vi "OpticsTester.vi"() -> ()   [LabVIEW 2024]
uses:
  <vilib>/SmarAct/SmarActCTL/SA_CTL.lvclass
  <vilib>/Platform/TimedLoop/XDataNode/timing_clust.ctl
  <vilib>/Platform/TimedLoop/XDataNode/nitl_modes.ctl
  <vilib>/Platform/TimedLoop/XDataNode/wakeup.ctl
  <vilib>/Utility/miscctls.llb/LVMajorAndMinorColorsTypeDef.ctl
  <vilib>/Analysis/1siggen.llb/Ramp Pattern by Delta.vi
  <vilib>/platform/TimedLoop/XDataNode/XDataNode.xnode
  <vilib>/Analysis/NI_AALBase.lvlib
  <userlib>/_OpenG.lib/time/time.llb/openg_time.lvlib
  <vilib>/Analysis/NI_AALPro.lvlib
  <vilib>/Platform/TimedLoop/XDataNode/XDNodeRunTimeDep.lvlib
  <instrlib>/Keithley 648X Series/Keithley 648X Series.lvlib
panel:
  in  "Measurement Time":dbl=6.0
  out "PicoAmmeter_VISA":refnum<visa-resource-name>
  in  "Oversample":i32=1000 min=1 max=4096
  out "Ref":dbl[](array[numeric])
  out "SweepData":dbl[][](array[numeric])
  in  "Exit":bool
  out "PositionerStatus":T1={"Moving"=FALSE, "CL Active"=FALSE, "Calibrating"=FALSE, "Referencing"=FALSE, "Delayed Move"=FALSE, "Sensor Present"=TRUE, "Is Calibrated"=TRUE, "Is Referenced"=TRUE, "End Stop"=FALSE, "Ranger Limit"=FALSE, "Following Limit"=FALSE, "Movement Fail"=FALSE, "Is Streaming"=FALSE, "Overload"=FALSE, "Over Temp"=FALSE, "Reference Mark"=FALSE, "Is Phased"=FALSE, "Positioner Fault"=FALSE, "Amplifier Enabled"=TRUE, "In Position"=FALSE, "Brake Enabled"=FALSE}
  out "ChannelState":i32=262368 format="%x"
  in  "Measurement Mode":T2(tab)=enum."Stage Calibration"
  in  "Device Locator":string(combo)="network:sn:MCS2-00005242"
  in  "findDevices":bool caption="Find Devices"
  in  "connect":bool
  out "connected":bool=TRUE
  out "Error Out":errorcluster
  in  "calibrate":bool
  in  "reference":bool
  in  "moveValue":i64=-10400000000 caption="Move Abs (µm)"
  in  "moveMode":u16(ring) caption="Move Mode" items=["CL_ABS", "CL_REL", "SCAN_ABS", "SCAN_REL", "STEP"]
  in  "move":bool
  in  "actuatorMode":enum32{"0", "1"}(radio)
  out "MCSChannel":i8
  out "Position (µm)":dbl=-7999576013.0
  in  "MoveStage":bool
  in  "Move To (mm)":dbl min=-13.5 max=13.5
  in  "Enable":bool=TRUE
  in  "Positioner\n Delay (ms)":u16(ring)=2 items=["1", "2", "5", "10", "20", "50", "100", "200", "500"]
  in  "Delay(mS)":u32=5
  out "Elapsed (ms)":dbl=6.0
  out "Waveform Chart":dbl(graph)=-7999.576013
  out "Peak-to-Peak (µm)":dbl=0.0026870000001508743 format="%^.4g"
  out "rms (µm)":dbl=-2.7284841053187847e-12 format="%^.4g"
  in  "Recalibrate":bool
  out "Calibration":cluster{"Array":dbl[], "Array":dbl[]}(graph)
  in  "Stage\nCal":dbl[][](array[numeric])=[[1020.0, -8440.0], [1100.0, -6120.0], [1200.0, -3330.0], [1300.0, -530.0], [1400.0, 2280.0], [1500.0, 5160.0], [1600.0, 8630.0]]
  out "slope":dbl
  out "intercept":dbl
  in  "Clear_Static":bool
  out "PhotoCurrent":dbl(graph)
  in  "Grid":bool
  in  "SetSample":bool
  in  "SetRef":bool
  in  "Dark Level":dbl
  out "End(nm)":dbl
  out "Start(nm)":dbl
  out "Sweep":cluster{"Ramp Pattern":dbl[], dbl[]}(graph)
  in  "Go":bool
  in  "Step(µm)":dbl=10.0 min=1.0 max=2000.0 step=1.0
  in  "Finish (mm)":dbl=-8.0 min=-12.0 max=12.0 step=1.0
  in  "Start (mm)":dbl=-12.0 min=-12.0 max=12.0 step=1.0
  in  "milliseconds\n to wait":u32 max=1000
  out "Elapsed(s)":dbl=32.049
  out "Cursor\nlambda":dbl
  out "samples":i32
  out "Step(nm)":dbl
  out "Reference":cluster{"Ramp Pattern":dbl[], dbl[]}(graph)
  out "Reflectance":cluster{"Ramp Pattern":dbl[], dbl[]}(graph)
  in  "Grid 2":bool
  in  "stop":bool
  out "Handle":refnum<class "SA_CTL.lvclass">
  out "exit":bool=TRUE
  # "Instrument uses optics breadboard for optics/LVF\n\nLVF stage driven by MCS2 controller\n\nCurrent monitoring thorugh Keithley 6845 Picoammeter"
  # "Stage \n(µm)"
  # "Wavelength\n (nm)"
  # "Reads photocurrent and displays against time"
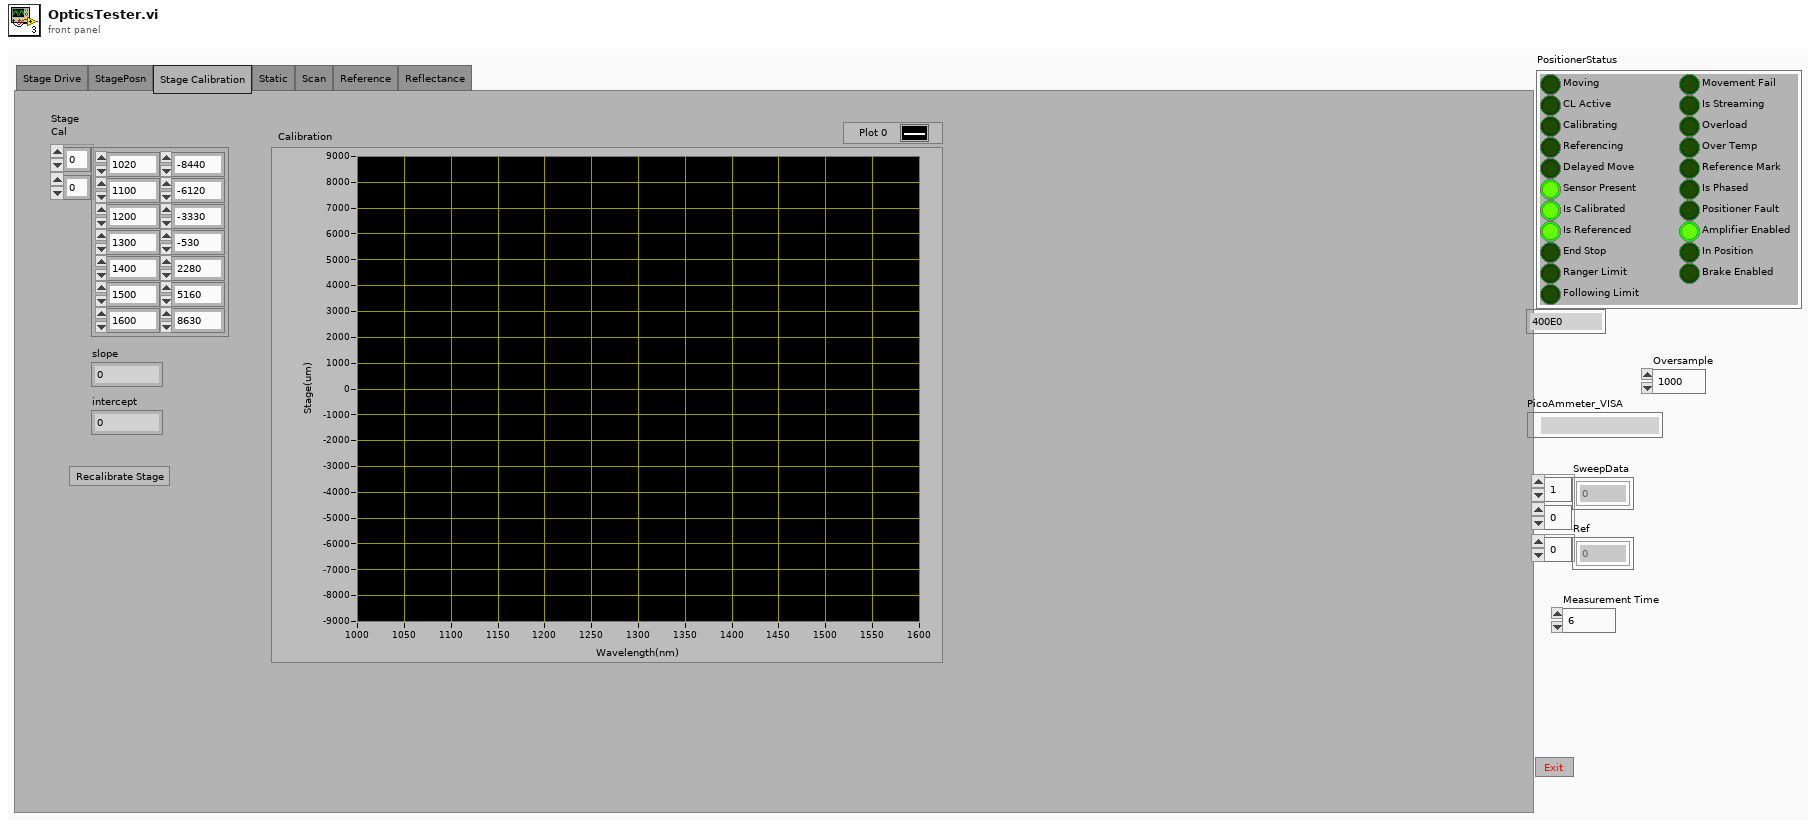
[diagram p1: front panel]
types:
  T1 = cluster{"Moving":bool, "CL Active":bool, "Calibrating":bool, "Referencing":bool, "Delayed Move":bool, "Sensor Present":bool, "Is Calibrated":bool, "Is Referenced":bool, "End Stop":bool, "Ranger Limit":bool, "Following Limit":bool, "Movement Fail":bool, "Is Streaming":bool, "Overload":bool, "Over Temp":bool, "Reference Mark":bool, "Is Phased":bool, "Positioner Fault":bool, "Amplifier Enabled":bool, "In Position":bool, "Brake Enabled":bool}
  T2 = enum32{"Stage Drive", "StagePosn", "Stage Calibration", "Static", "Scan", "Reference", "Reflectance"}
  T3 = typedef "XDNodeRunTimeDep.lvlib/timing_clust.ctl" = cluster{"Expected End [f-1]":u64, "Actual End [f-1]":u64, "Finished Late? [f-1]":bool, "Expected End [i-1]":u64, "Actual End [i-1]":u64, "Finished Late? [i-1]":bool, "Expected Start [i]":u64, "Actual Start [i]":u64, "Expected Start [f]":u64, "Actual Start [f]":u64, "Source Name":string, "Structure Name":string, "Period":i64, "Deadline":i64, "Offset":i64, "Start":i64, "Priority":i32, "Timeout":i32, "Mode":T4, "Wakeup Reason":T5, "Error":errorcluster, "Source Type":string, "Secondary Source Type":string, "Global End Time":u64, "Global Start Time":u64, "Frame Duration":u64, "Iteration Duration":u64, "Assigned CPU":i32, "I/O Scan Engine Mode":u32}
  T4 = typedef "XDNodeRunTimeDep.lvlib/nitl_modes.ctl" = enum32{"No Change", "Process missed periods, maintain original phase", "Discard missed periods, maintain original phase", "Process missed periods, ignore original phase", "Discard missed periods, ignore original phase"}
  T5 = typedef "XDNodeRunTimeDep.lvlib/wakeup.ctl" = enum32{"Normal", "Aborted", "Asynchronous wakeup", "Timing source error", "Timed loop error", "Timeout"}
  T6 = typedef "LVMajorAndMinorColorsTypeDef.ctl" = cluster{"Major Color":u32, "Minor Color":u32}
  T7 = cluster{"Boolean array[0]":bool, "Boolean array[1]":bool, "Boolean array[2]":bool, "Boolean array[3]":bool, "Boolean array[4]":bool, "Boolean array[5]":bool, "Boolean array[6]":bool, "Boolean array[7]":bool, "Boolean array[8]":bool, "Boolean array[9]":bool, "Boolean array[10]":bool, "Boolean array[11]":bool, "Boolean array[12]":bool, "Boolean array[13]":bool, "Boolean array[14]":bool, "Boolean array[15]":bool, "Boolean array[16]":bool, "Boolean array[17]":bool, "Boolean array[18]":bool, "Boolean array[19]":bool, "Boolean array[20]":bool}
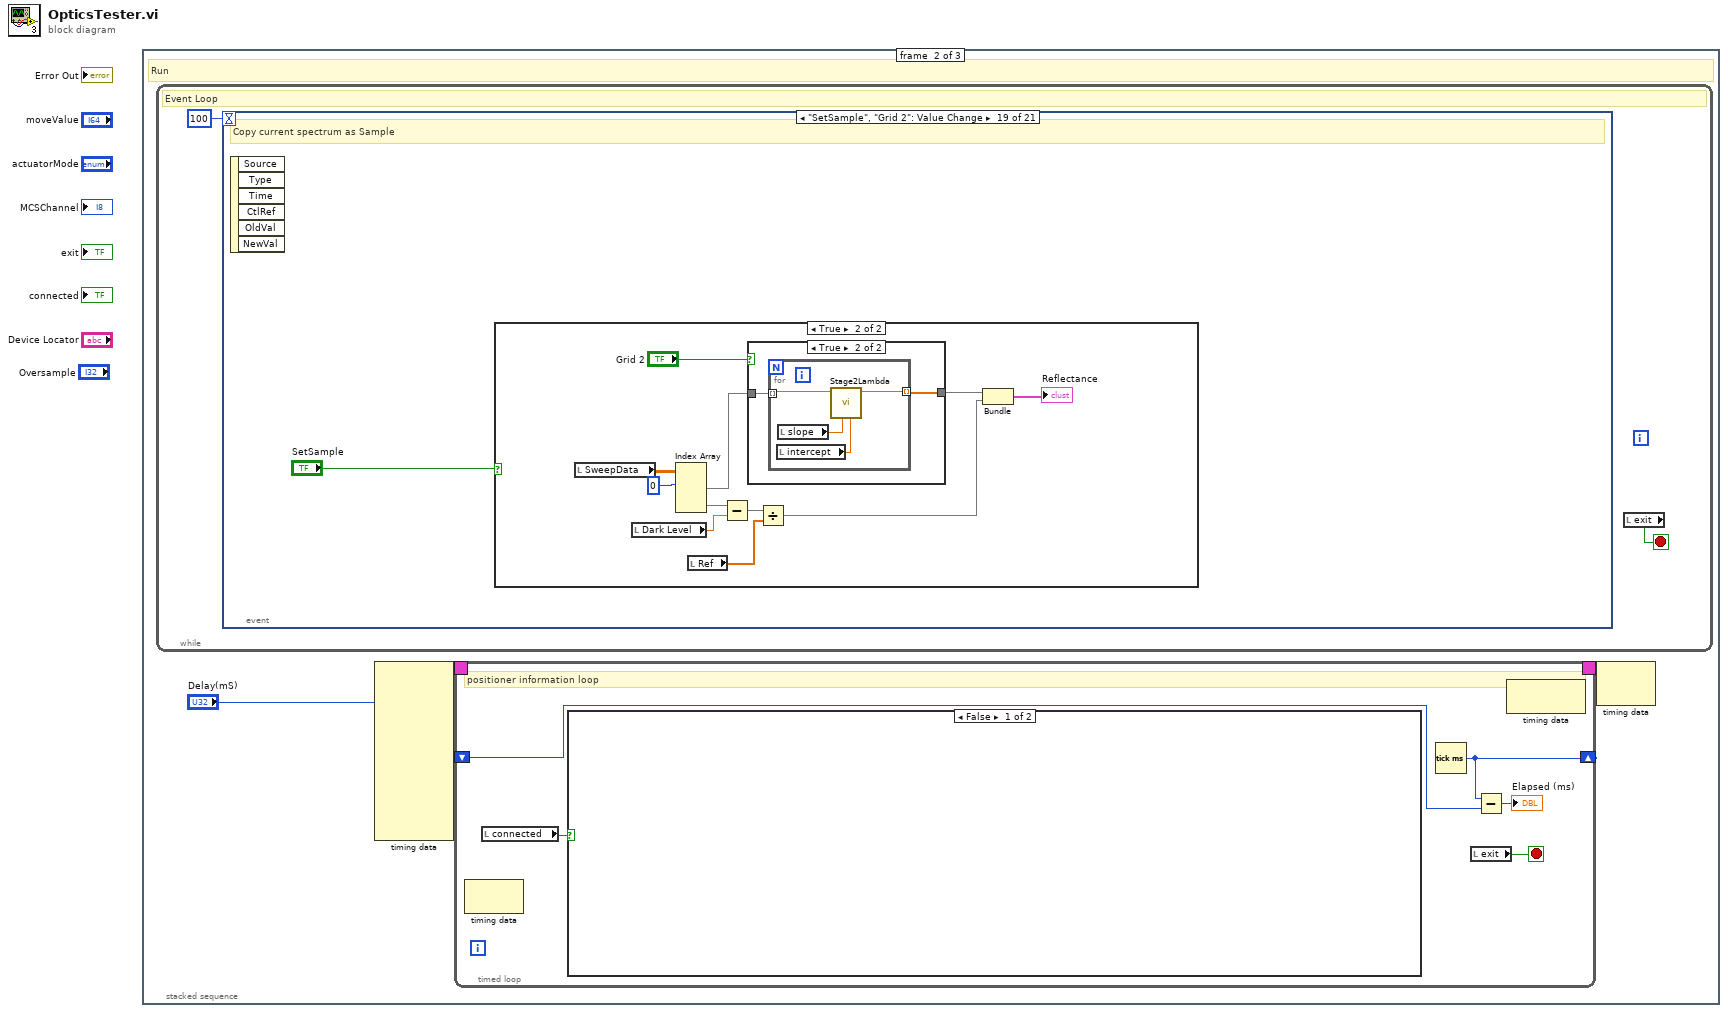
[diagram p0: block diagram]
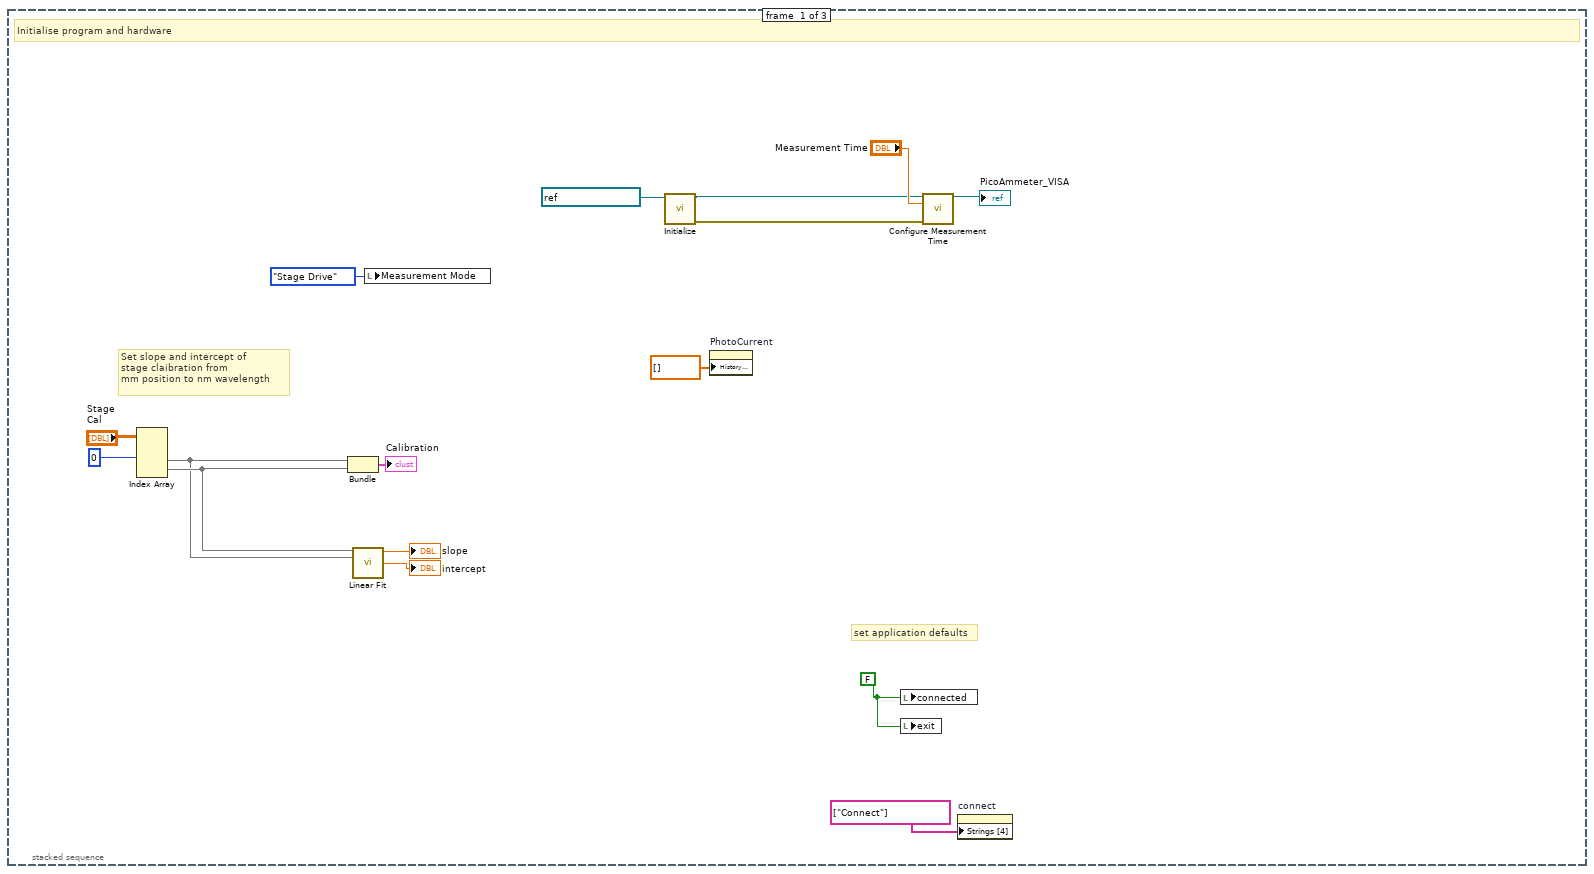
[diagram p2: hidden frame]
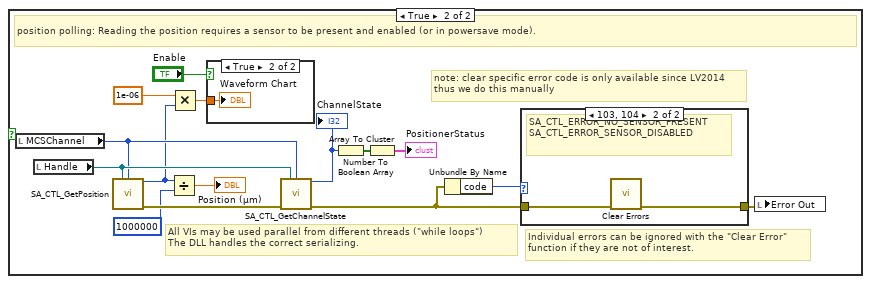
[diagram p3: hidden frame]
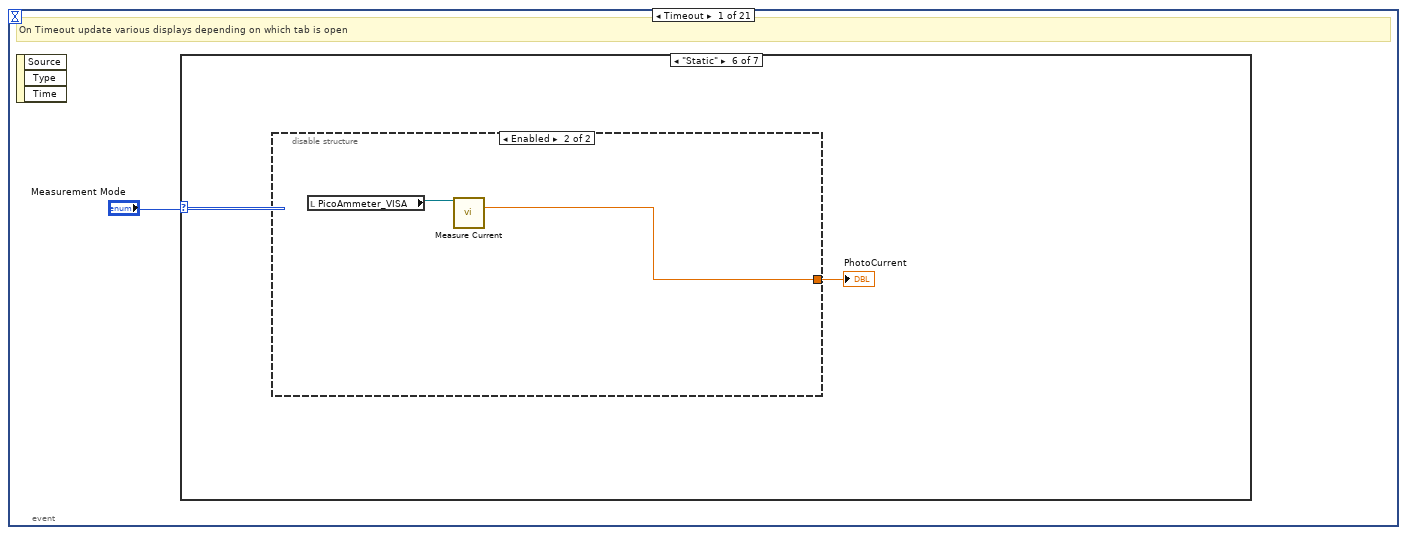
[diagram p6: hidden frame]
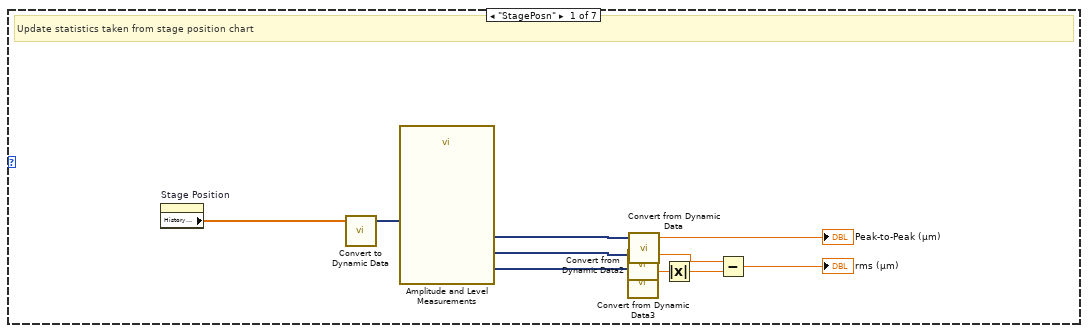
[diagram p7: hidden frame]
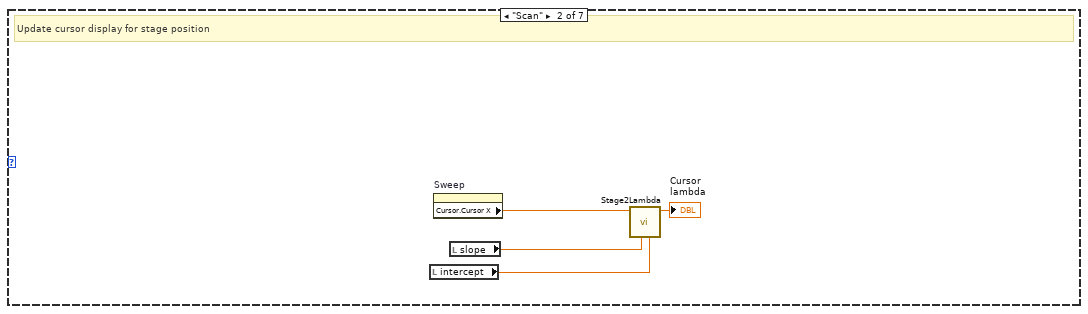
[diagram p8: hidden frame]
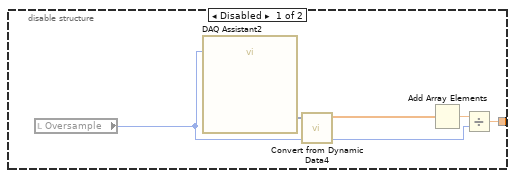
[diagram p12: hidden frame]
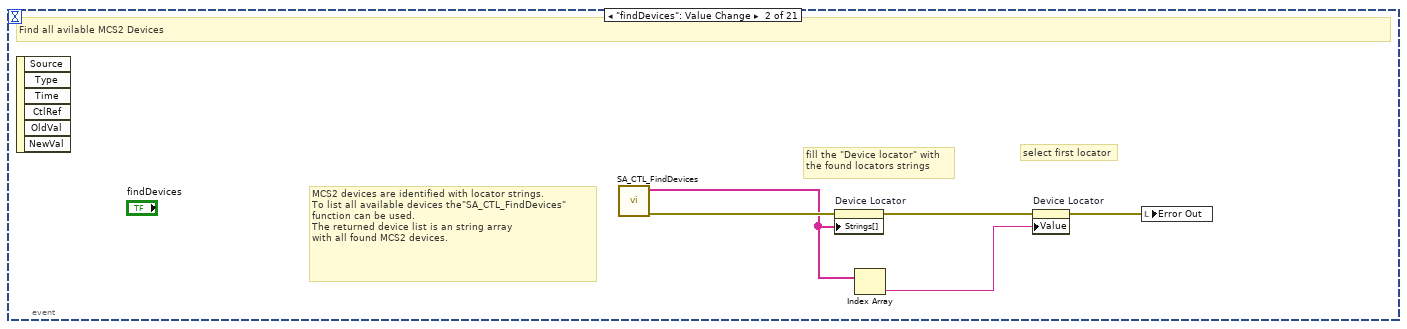
[diagram p14: hidden frame]
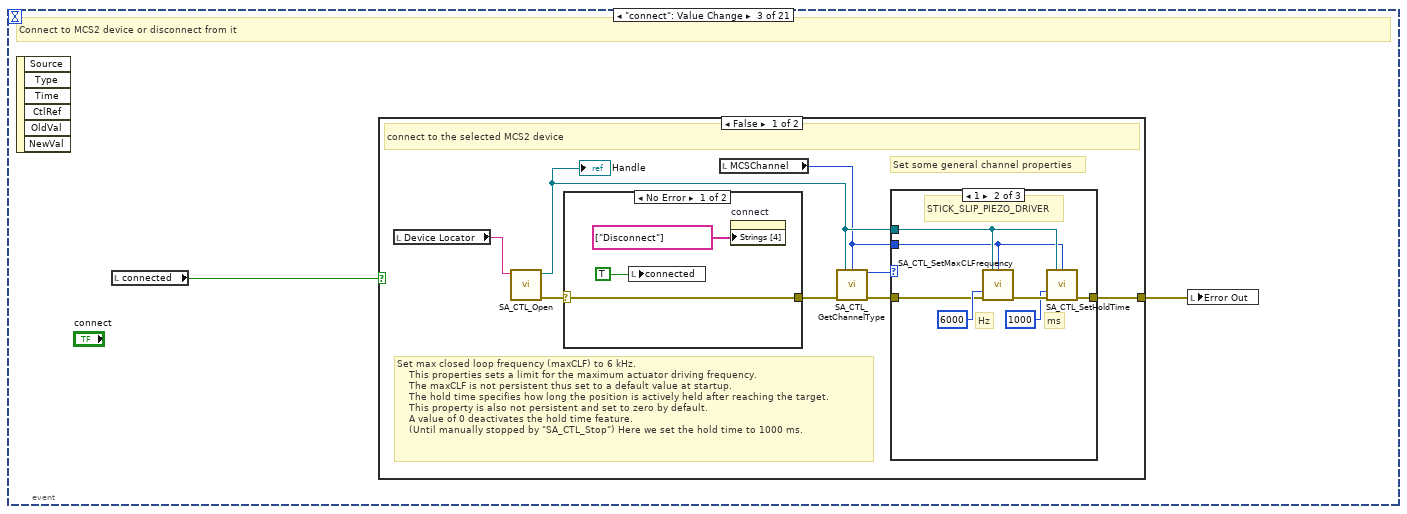
[diagram p15: hidden frame]
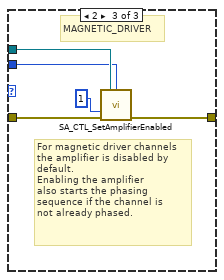
[diagram p17: hidden frame]
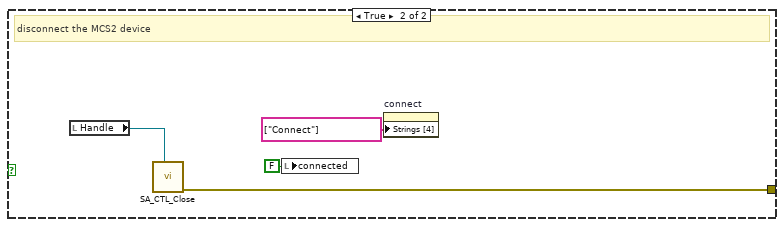
[diagram p19: hidden frame]
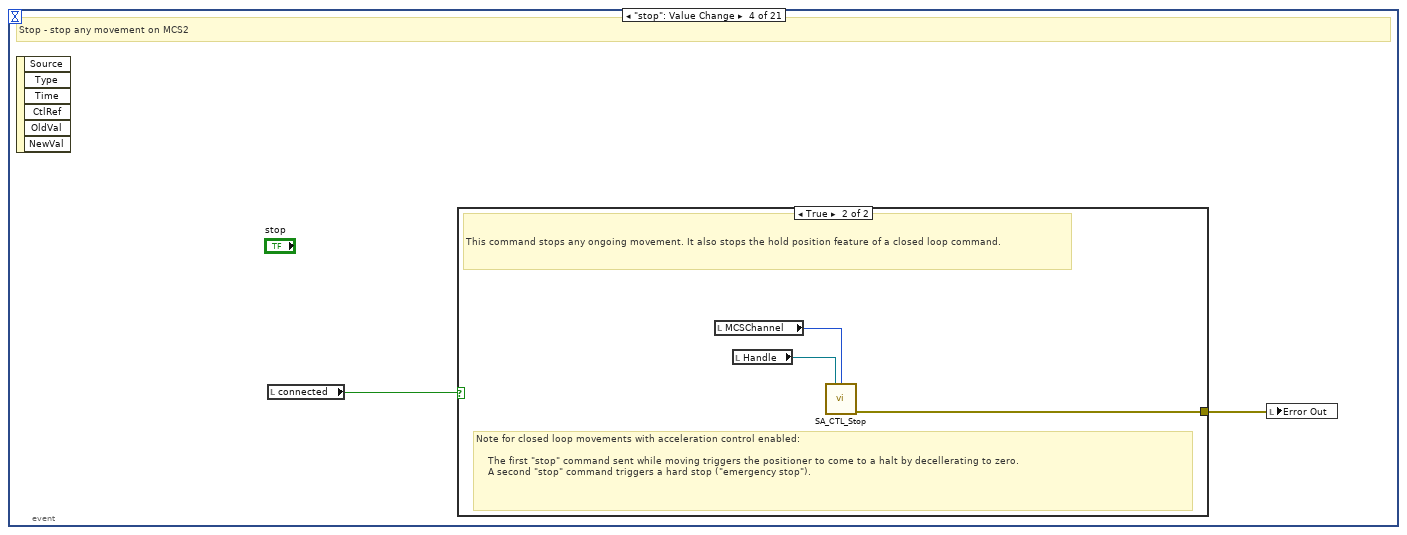
[diagram p20: hidden frame]
diagram:
  n1 = stacked-sequence {
    frame #0 {
      w15 = FALSE ("connected")
      # "Set slope and intercept of \nstage claibration from\nmm position to nm wavelength"
      # "set application defaults"
      # "Initialise program and hardware"
      n2 = Index Array(array="Stage\nCal", index (col) #1=0 ("disabled index (col)")) -> (element #1=w11:dbl[], element #2=w12:dbl[])  [unwired: 3 in]
      n3 = Bundle("Stage\nCal"=w11, "Stage\nCal"=w12) -> (→"Calibration":cluster{"Stage\nCal":dbl[], "Stage\nCal":dbl[]})  [unwired: 1 in]
      n4 = call <vilib>:"Linear Fit.vi"("Y"=w12, "X"=w11) -> ("slope"=→"slope":dbl, "intercept"=→"intercept":dbl)  [unwired: 9 in, 3 out]
      n5 = local write "Measurement Mode"(T2."Stage Drive" ("Measurement Mode")) -> ()
      n6 = call <instrlib>:"Initialize.vi"("VISA resource name"=refnum<visa-resource-name> "Picoammeter") -> ("error out"=w2:errorcluster, "VISA resource name out"=w3:refnum<visa-resource-name>)  [unwired: 9 in]
      n7 = property on="PhotoCurrent" class="WFChart (strict)"("History Data"=dbl[] []) -> ()  [unwired: 2 in, 2 out]
      n8 = local write "connected"(w15) -> ()
      n9 = local write "exit"(w15) -> ()
      n10 = call <instrlib>:"Configure Measurement Time.vi"("VISA resource name"=w3, "Measurement Time (6 PLC)"="Measurement Time", "error in (no error)"=w2) -> ("VISA resource name out"=→"PicoAmmeter_VISA":refnum<visa-resource-name>)  [unwired: 11 in, 1 out]
      n11 = property on="connect" class="Bool"("Strings [4]"=string[] ["Connect"]) -> ()  [unwired: 2 in, 2 out]
    }
    frame #1 {
      # "Run"
      n12 = while {
        stop <- w50 stop-if-true
        # "Event Loop"
        n13 = event shown="[18] \"SetSample\", \"Grid 2\": Value Change" {
          selector: _ -> [_ _ _ _ _ _ _ _ _ _ _ _ _ _ _ _ _ _ _ _ _]
          dyn-events: _ -> [_ _ _ _ _ _ _ _ _ _ _ _ _ _ _ _ _ _ _ _ _]
          timeout: 100 -> [_ _ _ _ _ _ _ _ _ _ _ _ _ _ _ _ _ _ _ _ _]
          event Timeout {
            # "On Timeout update various displays depending on which tab is open"
            n14 = event-data() -> ()  [unwired: 1 in, 3 out]
            n15 = case shown="\"Static\"" "Measurement Mode" {
              frame "StagePosn" {
                # "Update statistics taken from stage position chart"
                n16 = property on="Stage Position" class="WFChart (strict)"() -> ("History Data"=w62:dbl[])  [unwired: 2 in, 2 out]
                n17 = call "Convert to Dynamic Data"("Array"=w62) -> ("Dynamic Data Type"=w61:dynamicdata)  [unwired: 3 in]
                n18 = call "Amplitude and Level Measurements"("Signals"=w61) -> ("Mean (DC)"=w56:dynamicdata, "RMS"=w57:dynamicdata, "Peak to Peak"=w60:dynamicdata)  [unwired: 11 in, 1 out]
                n19 = call "Convert from Dynamic Data2"("Dynamic Data Type"=w57) -> ("Scalar"=w58:dbl)  [unwired: 3 in]
                n20 = call "Convert from Dynamic Data3"("Dynamic Data Type"=w56) -> ("Scalar"=w55:dbl)  [unwired: 3 in]
                n21 = call "Convert from Dynamic Data"("Dynamic Data Type"=w60) -> ("Scalar"=→"Peak-to-Peak (µm)":dbl)  [unwired: 3 in]
                n22 = Absolute Value(x=w55) -> (abs(x)=w53:dbl)
                n23 = Subtract(x=w58, y=w53) -> (x-y=→"rms (µm)":dbl)
              }
              frame "Scan" {
                # "Update cursor display for stage position"
                n24 = local read "intercept"() -> (w64:dbl)
                n25 = property on="Sweep" class="XYGraph (strict)"() -> ("Cursor.Cursor X"=w66:dbl)  [unwired: 2 in, 2 out]
                n26 = local read "slope"() -> (w65:dbl)
                n27 = call "Stage2Lambda.vi"("intercept"=w64, "slope"=w65, "Stage (mm)"=w66) -> ("lambda"=→"Cursor\nlambda":dbl)  [unwired: 8 in]
              }
              frame "Reference" {
              }
              frame "Reflectance" {
              }
              frame "Stage Calibration" {
              }
              frame "Static" {
                n28 = disable-structure shown="Enabled" {
                  disable-tunnel: [w69 w73] -> w67
                  frame Disabled {
                    n29 = local read "Oversample"() -> (w68:i32)
                    n30 = call "DAQ Assistant2"("number of samples"=w68) -> ("data"=w72:dynamicdata)  [unwired: 16 in, 2 out]
                    n31 = call "Convert from Dynamic Data4"("Dynamic Data Type"=w72) -> ("Array"=w71:dbl[])  [unwired: 3 in]
                    n32 = Add Array Elements(numeric array=w71) -> (sum=w70:dbl)
                    n33 = Divide(x=w70, y=w68) -> (x/y=w69:dbl)
                  }
                  frame Enabled {
                    n34 = local read "PicoAmmeter_VISA"() -> (w74:refnum<visa-resource-name>)
                    n35 = call <instrlib>:"Measure Current.vi"("VISA resource name"=w74) -> ("Measurement"=w73:dbl)  [unwired: 12 in, 2 out]
                  }
                }
                "PhotoCurrent" <- w67
              }
              frame "Stage Drive" {
              }
            }
          }
          event "findDevices": Value Change {
            # "select first locator"
            # "fill the \"Device locator\" with\nthe found locators strings"
            # "MCS2 devices are identified with locator strings.\nTo list all available devices the\"SA_CTL_FindDevices\"\nfunction can be used.\nThe returned device list is an string array \nwith all found MCS2 devices."
            # "Find all avilable MCS2 Devices"
            n36 = event-data() -> ()  [unwired: 1 in, 6 out]
            n37 = call <vilib>:"SA_CTL_FindDevices.vi"() -> ("error out"=w79:errorcluster, "devices"=w78:string[])  [unwired: 10 in]
            n38 = property on="Device Locator" class="CmbBox"(error in=w79, "Strings[]"=w78) -> (error out=w77:errorcluster)  [unwired: 1 in, 1 out]
            n39 = Index Array(array=w78) -> (element=w76:string)  [unwired: 1 in]
            n40 = property on="Device Locator" class="CmbBox"(error in=w77, "Value"=w76) -> (error out=w75:errorcluster)  [unwired: 1 in, 1 out]
            n41 = local write "Error Out"(w75) -> ()
          }
          event "connect": Value Change {
            # "Connect to MCS2 device or disconnect from it"
            n42 = event-data() -> ()  [unwired: 1 in, 6 out]
            n43 = local read "connected"() -> (w81:bool)
            n44 = case shown="False" w81 {
              tunnel: [w87 w107] -> w80
              frame False {
                # "Set max closed loop frequency (maxCLF) to 6 kHz.\n    This properties sets a limit for the maximum actuator driving frequency.\n    The maxCLF is not persistent thus set to a default value at startup.\n    The hold time specifies how long the position is actively held after reaching the target.\n    This property is also not persistent and set to zero by default.\n    A value of 0 deactivates the hold time feature.\n    (Until manually stopped by \"SA_CTL_Stop\") Here we set the hold time to 1000 ms."
                # "Set some general channel properties"
                # "connect to the selected MCS2 device"
                n45 = local read "Device Locator"() -> (w88:string)
                n46 = call <vilib>:"SA_CTL_Open.vi"("locator"=w88) -> ("error out"=w89:errorcluster, "SA_CTL_Handle"=w83:refnum<class "SA_CTL.lvclass">)  [unwired: 9 in]
                "Handle" <- w83
                n47 = case shown="No Error" w89 {
                  selector: w89 -> [w103 w106]
                  tunnel: [w103 w106] -> w86
                  frame No Error {
                    n48 = local write "connected"(TRUE ("connected")) -> ()
                    n49 = property on="connect" class="Bool"("Strings [4]"=string[] ["Disconnect"]) -> ()  [unwired: 2 in, 2 out]
                  }
                  frame Error {
                  }
                }
                n50 = local read "MCSChannel"() -> (w82:i8)
                n51 = call <vilib>:"SA_CTL_GetChannelType.vi"("SA_CTL_Handle"=w83, "channel"=w82, "error in (no error)"=w86) -> ("ChannelType"=w85:i32, "error out"=w84:errorcluster)  [unwired: 11 in]
                n52 = case shown="1" w85 {
                  tunnel: w83 -> [_ w94 w99]
                  tunnel: [w90 w93 w101] -> w87
                  tunnel: w82 -> [_ w92 w98]
                  tunnel: w84 -> [w90 w91 w102]
                  frame 0, Default {
                    # "unknown"
                  }
                  frame 1 {
                    # "Hz"
                    # "ms"
                    # "STICK_SLIP_PIEZO_DRIVER"
                    n53 = call <vilib>:"SA_CTL_SetMaxCLFrequency.vi"("SA_CTL_Handle"=w94, "channel"=w92, "MaxCLFrequency"=6000 ("MaxCLF"), "error in (no error)"=w91) -> ("error out"=w97:errorcluster)  [unwired: 11 in]
                    n54 = call <vilib>:"SA_CTL_SetHoldTime.vi"("SA_CTL_Handle"=w94, "channel"=w92, "HoldTime"=1000 ("MaxCLF"), "error in (no error)"=w97) -> ("error out"=w93:errorcluster)  [unwired: 11 in]
                  }
                  frame 2 {
                    # "For magnetic driver channels\nthe amplifier is disabled by\ndefault. \nEnabling the amplifier\nalso starts the phasing\nsequence if the channel is\nnot already phased."
                    # "MAGNETIC_DRIVER"
                    n55 = call <vilib>:"SA_CTL_SetAmplifierEnabled.vi"("SA_CTL_Handle"=w99, "channel"=w98, "AmplifierEnabled"=1, "error in (no error)"=w102) -> ("error out"=w101:errorcluster)  [unwired: 11 in]
                  }
                }
              }
              frame True {
                # "disconnect the MCS2 device"
                n56 = local read "Handle"() -> (w110:refnum<class "SA_CTL.lvclass">)
                n57 = call <vilib>:"SA_CTL_Close.vi"("SA_CTL_Handle"=w110) -> ("error out"=w107:errorcluster)  [unwired: 10 in]
                n58 = local write "connected"(FALSE ("connected")) -> ()
                n59 = property on="connect" class="Bool"("Strings [4]"=string[] ["Connect"]) -> ()  [unwired: 2 in, 2 out]
              }
            }
            n60 = local write "Error Out"(w80) -> ()
          }
          event "stop": Value Change {
            # "Stop - stop any movement on MCS2"
            n61 = event-data() -> ()  [unwired: 1 in, 6 out]
            n62 = local read "connected"() -> (w112:bool)
            n63 = case shown="True" w112 {
              tunnel: [_ w115] -> w111
              frame False {
              }
              frame True {
                # "Note for closed loop movements with acceleration control enabled:\n\n    The first \"stop\" command sent while moving triggers the positioner to come to a halt by decellerating to zero.\n    A second \"stop\" command triggers a hard stop (\"emergency stop\")."
                # "This command stops any ongoing movement. It also stops the hold position feature of a closed loop command."
                n64 = local read "MCSChannel"() -> (w113:i8)
                n65 = local read "Handle"() -> (w114:refnum<class "SA_CTL.lvclass">)
                n66 = call <vilib>:"SA_CTL_Stop.vi"("SA_CTL_Handle"=w114, "channel"=w113) -> ("error out"=w115:errorcluster)  [unwired: 13 in]
              }
            }
            n67 = local write "Error Out"(w111) -> ()
          }
          event "calibrate": Value Change {
            # "Calibratre MCS2"
            n68 = event-data() -> ()  [unwired: 1 in, 6 out]
            n69 = local read "connected"() -> (w117:bool)
            n70 = case shown="True" w117 {
              tunnel: [_ w122] -> w116
              frame False {
              }
              frame True {
                # "calibration options:\nstartDirection forward"
                # "Note that the function call (SA_CTL_Calibrate) returns immediatelly, without waiting for the movement to complete.\n    The \"SA_CTL_CH_STATE_BIT_CALIBRATING\" in the channel state can be monitored to determine the end of the calibration\n    sequence. \n \n WARNING\n    During the calibration sequence the positioner performs a movement of up to several mm, make sure to not start\n    the calibration near a mechanical endstop in order to ensure proper operation."
                # "The calibration sequence is used to increase the precision of the position calculation. This function should be called once for each\n    channel if the mechanical setup changes. (e.g. a different positioner was connected to the channel, the positioner type was set to a \n    different type) The calibration data will be saved to non-volatile memory, thus it is not necessaray to perform the calibration sequence\n    on each initialization. Note: the \"SA_CTL_CH_STATE_BIT_IS_CALIBRATED\" in the channel state can be used to determine\n    if valid calibration data is stored for the specific channel."
                n71 = local read "MCSChannel"() -> (w119:i8)
                n72 = local read "Handle"() -> (w120:refnum<class "SA_CTL.lvclass">)
                n73 = call <vilib>:"SA_CTL_SetCalibrationOptions.vi"("SA_CTL_Handle"=w120, "channel"=w119, "CalibrationOptions"=0 ("CalibrationMode")) -> ("error out"=w121:errorcluster)  [unwired: 12 in]
                n74 = call <vilib>:"SA_CTL_Calibrate.vi"("handle"=w120, "channel"=w119, "error in (no error)"=w121) -> ("error out"=w122:errorcluster)  [unwired: 12 in]
              }
            }
            n75 = local write "Error Out"(w116) -> ()
          }
          event "reference": Value Change {
            # "Find reference mark on stage"
            n76 = event-data() -> ()  [unwired: 1 in, 6 out]
            n77 = local read "connected"() -> (w124:bool)
            n78 = case shown="True" w124 {
              tunnel: [_ w133] -> w123
              frame False {
              }
              frame True {
                # "Note for Stick-Slip Driver:\nSetting the acceleration to zero \ndisables the acceleration control."
                # "The reference options specifies the behaviour of the find reference sequence. The reference flags can be ORed to build the \n    reference options. By default (options = 0) the positioner returns to the position of the reference mark.\n    Note: In contrast to previous controller systems this is not mandatory. The MCS2 controller is able to find the reference\n    position \"on-the-fly\". See the MCS2 Programmer Guide for a description of the different modes.\n    Note that the  function call (SA_CTL_Reference) returns immediatelly, without waiting for the movement to complete.\n    The \"SA_CTL_CH_STATE_BIT_REFERENCING\" in the channel state can be monitored to determine the end of the referencing\n    sequence.\n    Gere we use the \"autoZero\" option to set the position to zero after the reference position was found."
                # "Since the position sensors work on an incremental base, the referencing sequence is used to establish an absolute positioner \n    reference for the positioner after system startup.\n    Note: the \"SA_CTL_CH_STATE_BIT_IS_REFERENCED\" in the channel state can be used to to decide whether it is necessary\n    to perform the referencing sequence."
                n79 = local read "MCSChannel"() -> (w128:i8)
                n80 = local read "Handle"() -> (w129:refnum<class "SA_CTL.lvclass">)
                n81 = call <vilib>:"SA_CTL_SetReferencingOptions.vi"("SA_CTL_Handle"=w129, "channel"=w128, "ReferencingOptions"=0 ("CalibrationMode")) -> ("error out"=w131:errorcluster)  [unwired: 12 in]
                n82 = call <vilib>:"SA_CTL_SetMoveVelocity.vi"("SA_CTL_Handle"=w129, "channel"=w128, "MoveVelocity"=i64 1000000000 ("FindReferenceVelocity"), "error in (no error)"=w131) -> ("error out"=w132:errorcluster)  [unwired: 11 in]
                n83 = call <vilib>:"SA_CTL_SetMoveAcceleration.vi"("SA_CTL_Handle"=w129, "channel"=w128, "MoveAcceleration"=i64 10000000000 ("FindReferenceAcceleration"), "error in (no error)"=w132) -> ("error out"=w130:errorcluster)  [unwired: 11 in]
                n84 = call <vilib>:"SA_CTL_Reference.vi"("SA_CTL_Handle"=w129, "channel"=w128, "error in (no error)"=w130) -> ("error out"=w133:errorcluster)  [unwired: 12 in]
              }
            }
            n85 = local write "Error Out"(w123) -> ()
          }
          event "move": Value Change {
            # "Move stage"
            n86 = event-data() -> ()  [unwired: 1 in, 6 out]
            n87 = local read "connected"() -> (w137:bool)
            n88 = case shown="True" w137 {
              tunnel: [_ w148] -> w136
              frame False {
              }
              frame True {
                # "Note that the function call (SA_CTL_Move) returns immediatelly, without waiting for the movement to complete.\n    The \"SA_CTL_CH_STATE_BIT_ACTIVELY_MOVING\" and \"SA_CTL_CH_STATE_BIT_CLOSED_LOOP_ACTIVE\" in the channel state \n    can be monitored to determine the end of the movement."
                # "The move command instructs a positioner to perform a movement.\n    The given \"moveValue\" parameter is interpreted according to the previously configured move mode. It can be a position value\n    (in case of closed loop movement mode), a scan value (in case of scan move mode) or a number of steps (in case of step move mode)."
                n89 = local read "moveMode"() -> (w142:u16)
                n90 = local read "MCSChannel"() -> (w145:i8)
                n91 = local read "Handle"() -> (w140:refnum<class "SA_CTL.lvclass">)
                n92 = call <vilib>:"SA_CTL_SetMoveMode.vi"("SA_CTL_Handle"=w140, "channel"=w145, "MoveMode"=w142) -> ("error out"=w147:errorcluster)  [unwired: 12 in]
                n93 = case shown="0, 1, Default" w142 {
                  tunnel: w147 -> [w153 w159 w166]
                  tunnel: [w150 w156 w165] -> w146
                  tunnel: w145 -> [w152 w158 w162]
                  tunnel: [w152 w158 w162] -> w144
                  tunnel: w140 -> [w151 w157 w161]
                  tunnel: [w151 w157 w161] -> w143
                  frame 2, 3 {
                    # "scan velocity [in dac increments/s]"
                    n94 = call <vilib>:"SA_CTL_SetScanVelocity.vi"("SA_CTL_Handle"=w151, "channel"=w152, "ScanVelocity"=i64 65535, "error in (no error)"=w153) -> ("error out"=w150:errorcluster)  [unwired: 11 in]
                  }
                  frame 4 {
                    # "step amplitude [in dac incr.]\n0 to 65535 -> 0 to 100 V"
                    # "step frequency [in Hz]\nvalid range: 1 to 20000 Hz"
                    n95 = call <vilib>:"SA_CTL_SetStepFrequency.vi"("SA_CTL_Handle"=w157, "channel"=w158, "StepFrequency"=1000, "error in (no error)"=w159) -> ("error out"=w160:errorcluster)  [unwired: 11 in]
                    n96 = call <vilib>:"SA_CTL_SetStepAmplitude.vi"("SA_CTL_Handle"=w157, "channel"=w158, "StepAmplitude"=65535, "error in (no error)"=w160) -> ("error out"=w156:errorcluster)  [unwired: 11 in]
                  }
                  frame 0, 1, Default {
                    # "move velocity [in pm/s], move acceleration [in pm/s]\na value of 0 disables velocity/acceleration control\n(only Stick-Slip Drvier)"
                    n97 = call <vilib>:"SA_CTL_SetMoveVelocity.vi"("SA_CTL_Handle"=w161, "channel"=w162, "MoveVelocity"=i64 1000000000 ("FindReferenceVelocity"), "error in (no error)"=w166) -> ("error out"=w167:errorcluster)  [unwired: 11 in]
                    n98 = call <vilib>:"SA_CTL_SetMoveAcceleration.vi"("SA_CTL_Handle"=w161, "channel"=w162, "MoveAcceleration"=i64 1000000000 ("FindReferenceVelocity"), "error in (no error)"=w167) -> ("error out"=w165:errorcluster)  [unwired: 11 in]
                  }
                }
                n99 = local read "moveValue"() -> (w141:i64)
                n100 = Multiply(x=w141, y=i64 1000000) -> (x*y=w139:i64)
                n101 = call <vilib>:"SA_CTL_Move.vi"("moveValue"=w139, "SA_CTL_Handle"=w143, "channel"=w144, "error in (no error)"=w146) -> ("error out"=w148:errorcluster)  [unwired: 11 in]
              }
            }
            n102 = property on="move" class="Bool (strict)"(error in=w136, "Value"=FALSE ("move")) -> (error out=w135:errorcluster)  [unwired: 1 in, 1 out]
            n103 = local write "Error Out"(w135) -> ()
          }
          event "moveMode": Value Change {
            # "Put correct text in caption of MoveValue control"
            n104 = event-data() -> ()  [unwired: 1 in, 6 out]
            n105 = Index Array(array=string[] ["Move Abs (pm)", "Move Rel (pm)", "Move Value", "Move Value", "Move (steps)"], index="moveMode") -> (element=w169:string)
            n106 = property on="moveValue" class="DigNum (strict)"("Caption.Text"=w169) -> ()  [unwired: 2 in, 2 out]
          }
          event "actuatorMode": Value Change {
            # "Set Actuator Mode - Quiet/Normal"
            n107 = event-data() -> ("NewVal"=w171:enum32{"0", "1"})  [unwired: 1 in, 5 out]
            n108 = local read "connected"() -> (w173:bool)
            n109 = case shown="True" w173 {
              tunnel: [_ w176] -> w172
              tunnel: w171 -> [_ w174]
              frame False {
              }
              frame True {
                # "The actuator mode specifies the type of driving signal generation.\n        - normal mode (0) :    the control loop generates actuator driving signals with a maximum frequency limited to the max closed loop \n                                               frequency (maxCLF).\n        - quiet mode (1):        allows positioner movement with minimal noise emission.\n    Note that this property is not available for Magnetic Driver channels."
                n110 = local read "MCSChannel"() -> (w177:i8)
                n111 = local read "Handle"() -> (w175:refnum<class "SA_CTL.lvclass">)
                n112 = call <vilib>:"SA_CTL_SetActuatorMode.vi"("SA_CTL_Handle"=w175, "channel"=w177, "ActuatorMode"=w174) -> ("error out"=w176:errorcluster)  [unwired: 12 in]
              }
            }
            n113 = local write "Error Out"(w172) -> ()
          }
          event "Positioner\n Delay (ms)": Value Change {
            # "Sets delay between reading stage positioner"
            n114 = event-data() -> ()  [unwired: 1 in, 6 out]
            n115 = property on="Positioner\n Delay (ms)" class="Ring (strict)"() -> ("Strings []"=w181:string[])  [unwired: 2 in, 2 out]
            n116 = Index Array(array=w181, index="Positioner\n Delay (ms)") -> (element=w180:string)
            n117 = Decimal String To Number(string=w180) -> (number=w179:i32)  [unwired: 2 in, 1 out]
            n118 = local write "Delay(mS)"(w179) -> ()
          }
          event "Recalibrate": Value Change {
            # "Update slope and intercept for stageposn<=>lambda calculations from \"Stage Cal\" control"
            n119 = event-data() -> ()  [unwired: 1 in, 6 out]
            n120 = local read "Stage\nCal"() -> (w186:dbl[][])
            n121 = Index Array(array=w186, index (col) #1=0 ("disabled index (col)")) -> (element #1=w187:dbl[], element #2=w188:dbl[])  [unwired: 3 in]
            n122 = Bundle("Stage\nCal"=w187, "Stage\nCal"=w188) -> (w184:cluster{"Stage\nCal":dbl[], "Stage\nCal":dbl[]})  [unwired: 1 in]
            n123 = call <vilib>:"Linear Fit.vi"("Y"=w188, "X"=w187) -> ("slope"=w183:dbl, "intercept"=w182:dbl)  [unwired: 9 in, 3 out]
            n124 = local write "Calibration"(w184) -> ()
            n125 = local write "slope"(w183) -> ()
            n126 = local write "intercept"(w182) -> ()
          }
          event "Clear_Static": Value Change {
            n127 = event-data() -> ()  [unwired: 1 in, 6 out]
            n128 = property on="PhotoCurrent" class="WFChart (strict)"("History Data"=dbl[] []) -> ()  [unwired: 2 in, 2 out]
          }
          event "MoveStage": Value Change {
            # "1E9 converts mm to pm"
            # "Move stage in mm"
            n129 = event-data() -> ()  [unwired: 1 in, 6 out]
            n130 = local read "MCSChannel"() -> (w194:i8)
            n131 = local read "Handle"() -> (w190:refnum<class "SA_CTL.lvclass">)
            n132 = Multiply(x="Move To (mm)", y=1000000000.0) -> (x*y=w192:dbl)
            n133 = To Quad Integer(1:w192) -> (0:w191:i64)
            n134 = call <vilib>:"SA_CTL_Move.vi"("moveValue"=w191, "SA_CTL_Handle"=w190, "channel"=w194) -> ()  [unwired: 12 in, 1 out]
          }
          event "Go": Value Change {
            # "Initiate stage sweep"
            n135 = event-data() -> ()  [unwired: 1 in, 6 out]
            n136 = case shown="True" "Go" {
              frame False {
              }
              frame True {
                n137 = property on="Sweep" class="XYGraph (strict)"("ActXScl"=0 ("Active X Scale")) -> (error out=w201:errorcluster)  [unwired: 2 in, 1 out]
                n138 = local read "MCSChannel"() -> (w213:i8)
                n139 = local read "Handle"() -> (w212:refnum<class "SA_CTL.lvclass">)
                n140 = call <userlib>:"Tick Count (ms)__ogtk.vi"("error in (no error)"=w201) -> ("error out"=w209:errorcluster, "millisecond timer value"=w206:u32)  [unwired: 9 in]
                n141 = call <vilib>:"SA_CTL_SetMoveVelocity.vi"("SA_CTL_Handle"=w212, "channel"=w213, "MoveVelocity"=i64 0, "error in (no error)"=w209) -> ("error out"=w217:errorcluster)  [unwired: 11 in]
                n142 = Multiply(x=0.001, y="Step(µm)") -> (x*y=w219:dbl)
                n143 = call-poly <vilib>:"Ramp Pattern.vi"("start"="Start (mm)", "end"="Finish (mm)", "delta"=w219) -> ("samples"=→"samples":i32, "Ramp Pattern"=w210:dbl[])  [unwired: 6 in, 1 out]
                n144 = call <vilib>:"SA_CTL_SetMoveAcceleration.vi"("SA_CTL_Handle"=w212, "channel"=w213, "MoveAcceleration"=i64 0 ("FindReferenceVelocity"), "error in (no error)"=w217) -> ("error out"=w215:errorcluster)  [unwired: 11 in]
                n145 = for {
                  tunnel: w210 -> [w253] mode=indexing
                  tunnel: w213 -> [w249]
                  tunnel: w212 -> [w248]
                  tunnel: w215 -> [w245]
                  shift-right: [w242] -> w199
                  shift-left: dbl[] [] -> [w244]
                  tunnel: w210 -> [w241]
                  tunnel: [w225] -> w208
                  tunnel: [w241] -> w200
                  n146 = property on="Sweep" class="XYGraph (strict)"() -> (error out=w240:errorcluster, "ActXScl"=w238:i32)  [unwired: 2 in, 1 out]
                  n147 = Multiply(x=1000000000.0, y=w253) -> (x*y=w251:dbl)
                  n148 = call <vilib>:"SA_CTL_Move.vi"("moveValue"=w251, "SA_CTL_Handle"=w248, "channel"=w249, "error in (no error)"=w245) -> ("error out"=w250:errorcluster)  [unwired: 11 in]
                  n149 = property on="Sweep" class="XYGraph (strict)"(error in=w240, "ActXScl"=0 ("Active X Scale")) -> (error out=w239:errorcluster)  [unwired: 1 in, 1 out]
                  n150 = while {
                    tunnel: w250 -> [w261]
                    tunnel: w249 -> [w260]
                    tunnel: w248 -> [w259]
                    tunnel: [w255] -> w247
                    stop <- w257 stop-if-true
                    n151 = call <vilib>:"SA_CTL_GetChannelState.vi"("SA_CTL_Handle"=w259, "channel"=w260, "error in (no error)"=w261) -> ("ChannelState"=w258:i32, "error out"=w255:errorcluster)  [unwired: 11 in]
                    n152 = And(x=1, y=w258) -> (x .and. y?=w254:i32)
                    n153 = Equal To 0?(x=w254) -> (x = 0?=w257:bool)
                  }
                  n154 = property on="Sweep" class="XYGraph (strict)"(error in=w239) -> (error out=w237:errorcluster, "XScale.Maximum"=w234:dbl, "XScale.Minimum"=w232:dbl)  [unwired: 1 in, 1 out]
                  n155 = local read "intercept"() -> (w230:dbl)
                  n156 = local read "slope"() -> (w229:dbl)
                  n157 = call <userlib>:"Wait (ms)__ogtk.vi"("error in (no error)"=w247, "milliseconds to wait"="milliseconds\n to wait") -> ("error out"=w226:errorcluster)  [unwired: 8 in, 1 out]
                  n158 = property on="Sweep" class="XYGraph (strict)"(error in=w237, "ActXScl"=1 ("Active X Scale")) -> (error out=w235:errorcluster)  [unwired: 1 in, 1 out]
                  n159 = call "Stage2Lambda.vi"("intercept"=w230, "slope"=w229, "Stage (mm)"=w234) -> ("lambda"=w233:dbl)  [unwired: 8 in]
                  n160 = local read "PicoAmmeter_VISA"() -> (w223:refnum<visa-resource-name>)
                  n161 = call "Stage2Lambda.vi"("intercept"=w230, "slope"=w229, "Stage (mm)"=w232) -> ("lambda"=w231:dbl)  [unwired: 8 in]
                  n162 = call <instrlib>:"Measure Current.vi"("VISA resource name"=w223, "error in (no error)"=w226) -> ("Measurement"=w224:dbl, "error out"=w225:errorcluster)  [unwired: 11 in, 1 out]
                  n163 = property on="Sweep" class="XYGraph (strict)"(error in=w235, "XScale.Maximum"=w233, "XScale.Minimum"=w231) -> (error out=w236:errorcluster)  [unwired: 1 in, 1 out]
                  n164 = Build Array (concatenate)(w244, w224) -> (w242:dbl[])
                  n165 = Bundle("Ramp Pattern"=w241, w242) -> (→"Sweep":cluster{"Ramp Pattern":dbl[], dbl[]})  [unwired: 1 in]
                  n166 = property on="Sweep" class="XYGraph (strict)"(error in=w236, "ActXScl"=w238) -> ()  [unwired: 1 in, 2 out]
                }
                n167 = call <userlib>:"Tick Count (ms)__ogtk.vi"("error in (no error)"=w208) -> ("millisecond timer value"=w207:u32)  [unwired: 9 in, 1 out]
                n168 = Build Array(w200, w199) -> (→"SweepData":dbl[][])
                n169 = Subtract(x=w207, y=w206) -> (x-y=w205:u32)
                n170 = Multiply(x=0.001, y=w205) -> (x*y=→"Elapsed(s)":dbl)
              }
            }
          }
          event "Start (mm)", "Finish (mm)": Value Change {
            n171 = event-data() -> ()  [unwired: 1 in, 6 out]
            n172 = local read "slope"() -> (w266:dbl)
            n173 = local read "Start (mm)"() -> (w267:dbl)
            n174 = local read "intercept"() -> (w265:dbl)
            n175 = call "Stage2Lambda.vi"("intercept"=w265, "slope"=w266, "Stage (mm)"=w267) -> ("lambda"=→"Start(nm)":dbl)  [unwired: 8 in]
            n176 = local read "Finish (mm)"() -> (w264:dbl)
            n177 = call "Stage2Lambda.vi"("intercept"=w265, "slope"=w266, "Stage (mm)"=w264) -> ("lambda"=→"End(nm)":dbl)  [unwired: 8 in]
          }
          event "Grid": Value Change {
            # "Turn graph grid on/off"
            n178 = event-data() -> ()  [unwired: 1 in, 6 out]
            n179 = case shown="True" "Grid" {
              tunnel: [1 0] -> w272
              tunnel: [0 1] -> w271
              frame True {
              }
              frame False {
              }
            }
            n180 = property on="Sweep" class="XYGraph (strict)"() -> (error out=w270:errorcluster, "ActXScl"=w268:i32)  [unwired: 2 in, 1 out]
            n181 = property on="Sweep" class="XYGraph (strict)"(error in=w270, "ActXScl"=w272) -> (error out=w278:errorcluster)  [unwired: 1 in, 1 out]
            n182 = property on="Sweep" class="XYGraph (strict)"(error in=w278, "XScale.GridColors"=T6 {"Major Color"=0, "Minor Color"=0} ("X Scale.Grid Colors")) -> (error out=w276:errorcluster)  [unwired: 1 in, 1 out]
            n183 = property on="Sweep" class="XYGraph (strict)"(error in=w276, "ActXScl"=w271) -> (error out=w275:errorcluster)  [unwired: 1 in, 1 out]
            n184 = property on="Sweep" class="XYGraph (strict)"(error in=w275, "XScale.GridColors"=T6 {"Major Color"=10066176, "Minor Color"=5000192} ("X Scale.Grid Colors")) -> (error out=w269:errorcluster)  [unwired: 1 in, 1 out]
            n185 = property on="Sweep" class="XYGraph (strict)"(error in=w269, "ActXScl"=w268) -> ()  [unwired: 1 in, 2 out]
          }
          event "Step(µm)": Value Change {
            n186 = event-data() -> ("NewVal"=w285:dbl)  [unwired: 1 in, 5 out]
            n187 = local read "slope"() -> (w284:dbl)
            n188 = Divide(x=w285, y=w284) -> (x/y=→"Step(nm)":dbl)
          }
          event "SetRef": Value Change {
            # "Set Reference Spectrum"
            n189 = event-data() -> ()  [unwired: 1 in, 6 out]
            n190 = case shown="True" "SetRef" {
              frame False {
              }
              frame True {
                n191 = local read "SweepData"() -> (w293:dbl[][])
                n192 = Index Array(array=w293, index (row) #1=0 ("disabled index (col)")) -> (element #1=w290:dbl[], element #2=w292:dbl[])  [unwired: 3 in]
                n193 = Subtract(x=w292, y="Dark Level") -> (x-y=w289:dbl[])
                "Ref" <- w289
                n194 = Bundle("SweepData"=w290, w289) -> (→"Reference":cluster{"SweepData":dbl[], dbl[]})  [unwired: 1 in]
              }
            }
          }
          event "SetSample", "Grid 2": Value Change {
            # "Copy current spectrum as Sample"
            n195 = event-data() -> ()  [unwired: 1 in, 6 out]
            n196 = case shown="True" "SetSample" {
              frame False {
              }
              frame True {
                n197 = local read "SweepData"() -> (w305:dbl[][])
                n198 = local read "Dark Level"() -> (w303:dbl)
                n199 = Index Array(array=w305, index (row) #1=0 ("disabled index (col)")) -> (element #1=w300:dbl[], element #2=w304:dbl[])  [unwired: 3 in]
                n200 = local read "Ref"() -> (w301:dbl[])
                n201 = Subtract(x=w304, y=w303) -> (x-y=w302:dbl[])
                n202 = case shown="True" "Grid 2" {
                  tunnel: w300 -> [w306 w308]
                  tunnel: [w306 w307] -> w299
                  frame False {
                  }
                  frame True {
                    n203 = for {
                      tunnel: w308 -> [w312] mode=indexing
                      tunnel: [w309] -> w307 mode=indexing
                      n204 = local read "intercept"() -> (w310:dbl)
                      n205 = local read "slope"() -> (w311:dbl)
                      n206 = call "Stage2Lambda.vi"("intercept"=w310, "slope"=w311, "Stage (mm)"=w312) -> ("lambda"=w309:dbl)  [unwired: 8 in]
                    }
                  }
                }
                n207 = Divide(x=w302, y=w301) -> (x/y=w298:dbl[])
                n208 = Bundle("SweepData"=w299, w298) -> (→"Reflectance":cluster{"SweepData":dbl[], dbl[]})  [unwired: 1 in]
              }
            }
          }
          event "Exit": Value Change {
            # "If stage is connected, go to reference position and then exit"
            n209 = event-data() -> ()  [unwired: 1 in, 6 out]
            n210 = flat-sequence {
              frame #0 {
                n211 = local write "Measurement Mode"(T2."Stage Drive" ("Measurement Mode")) -> ()
              }
              frame #1 {
                n212 = local read "connected"() -> (w314:bool)
                n213 = case shown="True" w314 {
                  frame False {
                  }
                  frame True {
                    n214 = local read "MCSChannel"() -> (w316:i8)
                    n215 = local read "Handle"() -> (w315:refnum<class "SA_CTL.lvclass">)
                    n216 = call <vilib>:"SA_CTL_Move.vi"("moveValue"=i64 0, "SA_CTL_Handle"=w315, "channel"=w316) -> ("error out"=w317:errorcluster)  [unwired: 12 in]
                    n217 = while {
                      tunnel: w317 -> [w326]
                      tunnel: w316 -> [w325]
                      tunnel: w315 -> [w324]
                      tunnel: [w320] -> _
                      stop <- w322 stop-if-true
                      n218 = call <vilib>:"SA_CTL_GetChannelState.vi"("SA_CTL_Handle"=w324, "channel"=w325, "error in (no error)"=w326) -> ("ChannelState"=w323:i32, "error out"=w320:errorcluster)  [unwired: 11 in]
                      n219 = And(x=1, y=w323) -> (x .and. y?=w319:i32)
                      n220 = Equal To 0?(x=w319) -> (x = 0?=w322:bool)
                    }
                  }
                }
              }
              frame #2 {
                n221 = local write "exit"(TRUE) -> ()
              }
            }
          }
          event Panel Close? {
            # "Discard \"Panel Close?\" event\n\nto leave program through\n graceful route"
            # "NOTE:\nMake sure not to use the red \"Abort Execution\" button in the\nLabVIEW menu to abort the application execution.\nDoing so will not close the device connection with the consequence that\na re-open after the next application start will fail."
            # "\"Panel Close\" (\"X\") was clicked by the user:\nWe discard the close command and set an \"exit\" flag. This gives us the change to proper disconnect the device and clean up the application before closing the window."
            # "Trap \"Panel Close\" instruction and exit program gracefully"
            n222 = event-data() -> ()  [unwired: 1 in, 4 out]
            n223 = local write "exit"(TRUE ("exit")) -> ()
            n224 = event-data("Discard?"=TRUE) -> ()  [unwired: 1 in, 1 out]
          }
        }
        n225 = local read "exit"() -> (w50:bool)
      }
      n226 = node-c288("Delay(mS)") -> (w19:T3)  [unwired: 9 in]
      n227 = timed-loop {
        shift-right: [w22] -> _
        shift-left: _ -> [w21]
        timing: w19 -> [_]
        timing-out: [_] -> w18
        stop <- w24 stop-if-true
        # "positioner information loop"
        n228 = node-c288() -> ()  [unwired: 1 in, 1 out]
        n229 = local read "connected"() -> (w23:bool)
        n230 = case shown="False" w23 {
          frame False {
          }
          frame True {
            # "note: clear specific error code is only available since LV2014\nthus we do this manually"
            # "Individual errors can be ignored with the \"Clear Error\"\nfunction if they are not of interest."
            # "All VIs may be used parallel from different threads (\"while loops\")\nThe DLL handles the correct serializing."
            # "position polling: Reading the position requires a sensor to be present and enabled (or in powersave mode)."
            n231 = local read "MCSChannel"() -> (w36:i8)
            n232 = local read "Handle"() -> (w37:refnum<class "SA_CTL.lvclass">)
            n233 = call <vilib>:"SA_CTL_GetPosition.vi"("SA_CTL_Handle"=w37, "channel"=w36) -> ("Position"=w35:i64, "error out"=w39:errorcluster)  [unwired: 12 in]
            n234 = Divide(x=w35, y=i64 1000000 ("x")) -> (x/y=→"Position (µm)":dbl)
            n235 = Multiply(x=1e-06, y=w35) -> (x*y=w34:dbl)
            n236 = case shown="True" "Enable" {
              tunnel: w34 -> [_ w42]
              frame False {
              }
              frame True {
                "Waveform Chart" <- w42
              }
            }
            n237 = call <vilib>:"SA_CTL_GetChannelState.vi"("SA_CTL_Handle"=w37, "channel"=w36, "error in (no error)"=w39) -> ("ChannelState"=w32:i32, "error out"=w38:errorcluster)  [unwired: 11 in]
            "ChannelState" <- w32
            n238 = Number To Boolean Array(number=w32) -> (Boolean array=w31:bool[])
            n239 = Array To Cluster(array=w31) -> (cluster=→"PositionerStatus":T7)
            n240 = Unbundle By Name(w38) -> ("code"=w40:i32)
            n241 = case shown="103, 104" w40 {
              tunnel: w38 -> [w43 w45]
              tunnel: [w43 w44] -> w41
              frame Default {
              }
              frame 259, 260 {
                # "SA_CTL_ERROR_NO_SENSOR_PRESENT\nSA_CTL_ERROR_SENSOR_DISABLED"
                n242 = call <vilib>:"Clear Errors.vi"("error in (no error)"=w45) -> ("error out"=w44:errorcluster)  [unwired: 5 in, 1 out]
              }
            }
            n243 = local write "Error Out"(w41) -> ()
          }
        }
        n244 = Tick Count (ms)() -> (millisecond timer value=w22:u32)
        n245 = local read "exit"() -> (w24:bool)
        n246 = Subtract(x=w22, y=w21) -> (x-y=→"Elapsed (ms)":u32)
        n247 = node-c288() -> ()  [unwired: 1 in, 1 out]
      }
      n248 = node-c288(w18) -> ()  [unwired: 1 out]
    }
    frame #2 {
      # "Cleanup and Shutdown"
      n249 = local read "connected"() -> (w331:bool)
      n250 = case shown="True" w331 {
        frame False {
        }
        frame True {
          # "always make sure to close the connection\nto the device before quitting the program"
          n251 = local read "Handle"() -> (w332:refnum<class "SA_CTL.lvclass">)
          n252 = call <vilib>:"SA_CTL_Close.vi"("SA_CTL_Handle"=w332) -> ()  [unwired: 10 in, 1 out]
        }
      }
      n253 = local read "PicoAmmeter_VISA"() -> (w330:refnum<visa-resource-name>)
      n254 = call <instrlib>:"Close.vi"("VISA resource name"=w330) -> ()  [unwired: 10 in, 1 out]
    }
  }
